vi "HandleObservationSync_003.vi"(8 "error in (no error)":errorcluster, 11 "S4GUI in":refnum<class "S4GUI.lvclass">) -> (0 "error out":errorcluster, 3 "S4GUI out":refnum<class "S4GUI.lvclass">)   [LabVIEW 2018, in "S4GUI.lvclass"] (continued)
          n499 = call-dynamic "Read Channel.vi"("error in (no error)"=w1285, "Acquisition in"=w1286) -> ("error out"=w1268:errorcluster, "Channel.lvclass"=w1267:refnum<class "Channel.lvclass">, "Acquisition out"=w1295:refnum<class "Acquisition.lvclass">)  [unwired: 7 in]
          n500 = call-dynamic "Read Interface.vi"("error in (no error)"=w1268, "Channel in"=w1267) -> ("error out"=w1266:errorcluster, "Interface.lvclass"=w1272:refnum<class "Interface.lvclass">, "Channel out"=w1271:refnum<class "Channel.lvclass">)  [unwired: 7 in]
          n501 = call-dynamic "Get CCD_Config.vi"("error in (no error)"=w1266, "Interface in"=w1272) -> ("error out"=w1279:errorcluster, "output cluster"=w1281:T1, "Interface out"=w1278:refnum<class "Interface.lvclass">)  [unwired: 7 in]
          n502 = Bundle By Name(cluster=w1281, "TRIGGER_MODE"=w1280) -> (w1277:T1)
          n503 = call-dynamic "Set CCD_Config.vi"("error in (no error)"=w1279, "input cluster"=w1277, "Interface in"=w1278) -> ("error out"=w1275:errorcluster, "Interface out"=w1273:refnum<class "Interface.lvclass">)  [unwired: 7 in]
          n504 = Flatten To String(anything=w1277, error in (no error)=w1275) -> (data string=w1276:string, error out=w1274:errorcluster)  [unwired: 2 in, 1 out]
          n505 = call "Write flatted cluster.vi"("error in (no error)"=w1274, "flatted cluster"=w1276, "Interface in"=w1273) -> ("error out"=w1269:errorcluster, "Interface out"=w1270:refnum<class "Interface.lvclass">)  [unwired: 7 in]
          n506 = Increment(x=w1306) -> (x+1=w1305:u32)
          n507 = call-dynamic "Write Interface.vi"("error in (no error)"=w1269, "Interface.lvclass"=w1270, "Channel in"=w1271) -> ("error out"=w1265:errorcluster, "Channel out"=w1264:refnum<class "Channel.lvclass">)  [unwired: 7 in]
          n508 = call-dynamic "Read State Machine.vi"("error in (no error)"=w1265, "Device in"=w1264) -> ("error out"=w1292:errorcluster, "State Machine.lvclass"=w1294:refnum<class "State Machine.lvclass">, "Device out"=w1290:refnum<class "Channel.lvclass">)  [unwired: 7 in]
          n509 = call "Next State.vi"("error in (no error)"=w1292, "New_State"=60, "State Machine in"=w1294) -> ("error out"=w1287:errorcluster, "State Machine out"=w1288:refnum<class "State Machine.lvclass">)  [unwired: 7 in]
          n510 = call-dynamic "Write State Machine.vi"("error in (no error)"=w1287, "State Machine.lvclass"=w1288, "Device in"=w1290) -> ("error out"=w1289:errorcluster, "Device out"=w1291:refnum<class "Channel.lvclass">)  [unwired: 7 in]
          n511 = call-dynamic "Write Channel.vi"("error in (no error)"=w1289, "Channel.lvclass"=w1291, "Acquisition in"=w1295) -> ("error out"=w1282:errorcluster, "Acquisition out"=w1283:refnum<class "Acquisition.lvclass">)  [unwired: 7 in]
          n512 = call-dynamic "Write AcquisitionA.vi"("error in (no error)"=w1282, "Acquisition.lvclass"=w1283, "S4ACS_GUI in"=w1284) -> ("error out"=w1297:errorcluster, "S4ACS_GUI out"=w1296:refnum<class "S4GUI.lvclass">)  [unwired: 7 in]
          n513 = Bundle By Name(cluster=w1296, "Obs_state"=w1305) -> (w1304:refnum<class "S4GUI.lvclass">)
        }
        frame 254 {
          # "Espera terminar a execução do comando atual \nantes de ir ao proximo passo da Observação."
          n514 = call-dynamic "Read AcquisitionA.vi"("error in (no error)"=w1326, "S4ACS_GUI in"=w1327) -> ("error out"=w1332:errorcluster, "Acquisition.lvclass"=w1333:refnum<class "Acquisition.lvclass">, "S4ACS_GUI out"=w1329:refnum<class "S4GUI.lvclass">)  [unwired: 7 in]
          n515 = call-dynamic "Read Channel.vi"("error in (no error)"=w1332, "Acquisition in"=w1333) -> ("error out"=w1324:errorcluster, "Channel.lvclass"=w1323:refnum<class "Channel.lvclass">, "Acquisition out"=w1331:refnum<class "Acquisition.lvclass">)  [unwired: 7 in]
          n516 = call-dynamic "Read State Machine.vi"("error in (no error)"=w1324, "Device in"=w1323) -> ("error out"=w1315:errorcluster, "State Machine.lvclass"=w1317:refnum<class "State Machine.lvclass">, "Device out"=w1321:refnum<class "Channel.lvclass">)  [unwired: 7 in]
          n517 = call-dynamic "Read State.vi"("error in (no error)"=w1315, "State Machine in"=w1317) -> ("error out"=w1314:errorcluster, "State"=w1311:i32, "State Machine out"=w1316:refnum<class "State Machine.lvclass">)  [unwired: 7 in]
          n518 = Equal To 0?(x=w1311) -> (x = 0?=w1313:bool)
          n519 = call-dynamic "Write State Machine.vi"("error in (no error)"=w1314, "State Machine.lvclass"=w1316, "Device in"=w1321) -> ("error out"=w1320:errorcluster, "Device out"=w1322:refnum<class "Channel.lvclass">)  [unwired: 7 in]
          n520 = call-dynamic "Write Channel.vi"("error in (no error)"=w1320, "Channel.lvclass"=w1322, "Acquisition in"=w1331) -> ("error out"=w1328:errorcluster, "Acquisition out"=w1330:refnum<class "Acquisition.lvclass">)  [unwired: 7 in]
          n521 = disable-structure shown="Enabled" {
            disable-tunnel: [u32 299 ("t") w1335] -> w1310
            disable-tunnel: w1309 -> [_ w1336]
            frame Disabled {
            }
            frame Enabled {
              n522 = Increment(x=w1336) -> (x+1=w1335:u32)
            }
          }
          n523 = Select(t=w1310, s=w1313, f=w1309) -> (s? t:f=w1312:u32)
          n524 = call-dynamic "Write AcquisitionA.vi"("error in (no error)"=w1328, "Acquisition.lvclass"=w1330, "S4ACS_GUI in"=w1329) -> ("error out"=w1325:errorcluster, "S4ACS_GUI out"=w1319:refnum<class "S4GUI.lvclass">)  [unwired: 7 in]
          n525 = Bundle By Name(cluster=w1319, "Obs_state"=w1312) -> (w1318:refnum<class "S4GUI.lvclass">)
        }
        frame 255 {
          n526 = call "Read AcquisitionB.vi"("error in (no error)"=w1347, "S4ACS_GUI in"=w1348) -> ("error out"=w1340:errorcluster, "Acquisition.lvclass"=w1341:refnum<class "Acquisition.lvclass">, "S4ACS_GUI out"=w1350:refnum<class "S4GUI.lvclass">)  [unwired: 7 in]
          n527 = call "Read connection.vi"("error in (no error)"=w1340, "Server in"=w1341) -> ("error out"=w1339:errorcluster, "connection"=w1337:bool, "Server out"=w1338:refnum<class "Acquisition.lvclass">)  [unwired: 7 in]
          n528 = case shown="False" w1337 {
            tunnel: w1338 -> [w1358 w1378]
            tunnel: w1339 -> [w1357 w1377]
            tunnel: [w1358 w1375] -> w1351
            tunnel: [w1357 w1374] -> w1349
            tunnel: w1344 -> [w1356 w1367]
            tunnel: [w1352 w1366] -> w1343
            frame False {
              n529 = Increment(x=w1356) -> (x+1=w1355:u32)
              n530 = Increment(x=w1355) -> (x+1=w1354:u32)
              n531 = Increment(x=w1354) -> (x+1=w1353:u32)
              n532 = Increment(x=w1353) -> (x+1=w1352:u32)
            }
            frame True {
              # "configura o canal,\nmas não dispara\na exposicao."
              n533 = call-dynamic "Read Channel.vi"("error in (no error)"=w1377, "Acquisition in"=w1378) -> ("error out"=w1363:errorcluster, "Channel.lvclass"=w1365:refnum<class "Channel.lvclass">, "Acquisition out"=w1376:refnum<class "Acquisition.lvclass">)  [unwired: 7 in]
              n534 = call-dynamic "Write expose.vi"("error in (no error)"=w1363, "expose"=FALSE, "Channel in"=w1365) -> ("error out"=w1362:errorcluster, "Channel out"=w1364:refnum<class "Channel.lvclass">)  [unwired: 7 in]
              n535 = call-dynamic "Read State Machine.vi"("error in (no error)"=w1362, "Device in"=w1364) -> ("error out"=w1371:errorcluster, "State Machine.lvclass"=w1373:refnum<class "State Machine.lvclass">, "Device out"=w1369:refnum<class "Channel.lvclass">)  [unwired: 7 in]
              n536 = call "Next State.vi"("error in (no error)"=w1371, "New_State"=1, "State Machine in"=w1373) -> ("error out"=w1359:errorcluster, "State Machine out"=w1360:refnum<class "State Machine.lvclass">)  [unwired: 7 in]
              n537 = Increment(x=w1367) -> (x+1=w1366:u32)
              n538 = call-dynamic "Write State Machine.vi"("error in (no error)"=w1359, "State Machine.lvclass"=w1360, "Device in"=w1369) -> ("error out"=w1368:errorcluster, "Device out"=w1370:refnum<class "Channel.lvclass">)  [unwired: 7 in]
              n539 = call-dynamic "Write Channel.vi"("error in (no error)"=w1368, "Channel.lvclass"=w1370, "Acquisition in"=w1376) -> ("error out"=w1374:errorcluster, "Acquisition out"=w1375:refnum<class "Acquisition.lvclass">)  [unwired: 7 in]
            }
          }
          n540 = call "Write AcquisitionB.vi"("error in (no error)"=w1349, "Acquisition.lvclass"=w1351, "S4ACS_GUI in"=w1350) -> ("error out"=w1346:errorcluster, "S4ACS_GUI out"=w1345:refnum<class "S4GUI.lvclass">)  [unwired: 7 in]
          n541 = Bundle By Name(cluster=w1345, "Obs_state"=w1343) -> (w1342:refnum<class "S4GUI.lvclass">)
        }
        frame 256 {
          # "Espera terminar a execução do comando atual \nantes de ir ao proximo passo da Observação."
          n542 = call "Read AcquisitionB.vi"("error in (no error)"=w1396, "S4ACS_GUI in"=w1397) -> ("error out"=w1402:errorcluster, "Acquisition.lvclass"=w1403:refnum<class "Acquisition.lvclass">, "S4ACS_GUI out"=w1399:refnum<class "S4GUI.lvclass">)  [unwired: 7 in]
          n543 = call-dynamic "Read Channel.vi"("error in (no error)"=w1402, "Acquisition in"=w1403) -> ("error out"=w1394:errorcluster, "Channel.lvclass"=w1393:refnum<class "Channel.lvclass">, "Acquisition out"=w1401:refnum<class "Acquisition.lvclass">)  [unwired: 7 in]
          n544 = call-dynamic "Read State Machine.vi"("error in (no error)"=w1394, "Device in"=w1393) -> ("error out"=w1385:errorcluster, "State Machine.lvclass"=w1387:refnum<class "State Machine.lvclass">, "Device out"=w1391:refnum<class "Channel.lvclass">)  [unwired: 7 in]
          n545 = call-dynamic "Read State.vi"("error in (no error)"=w1385, "State Machine in"=w1387) -> ("error out"=w1384:errorcluster, "State"=w1381:i32, "State Machine out"=w1386:refnum<class "State Machine.lvclass">)  [unwired: 7 in]
          n546 = call-dynamic "Write State Machine.vi"("error in (no error)"=w1384, "State Machine.lvclass"=w1386, "Device in"=w1391) -> ("error out"=w1390:errorcluster, "Device out"=w1392:refnum<class "Channel.lvclass">)  [unwired: 7 in]
          n547 = call-dynamic "Write Channel.vi"("error in (no error)"=w1390, "Channel.lvclass"=w1392, "Acquisition in"=w1401) -> ("error out"=w1398:errorcluster, "Acquisition out"=w1400:refnum<class "Acquisition.lvclass">)  [unwired: 7 in]
          n548 = Equal To 0?(x=w1381) -> (x = 0?=w1383:bool)
          n549 = disable-structure shown="Enabled" {
            disable-tunnel: [u32 299 ("t") w1405] -> w1379
            disable-tunnel: w1380 -> [_ w1408]
            frame Disabled {
            }
            frame Enabled {
              n550 = Increment(x=w1408) -> (x+1=w1407:u32)
              n551 = Increment(x=w1407) -> (x+1=w1406:u32)
              n552 = Increment(x=w1406) -> (x+1=w1405:u32)
            }
          }
          n553 = Select(t=w1379, s=w1383, f=w1380) -> (s? t:f=w1382:u32)
          n554 = call "Write AcquisitionB.vi"("error in (no error)"=w1398, "Acquisition.lvclass"=w1400, "S4ACS_GUI in"=w1399) -> ("error out"=w1395:errorcluster, "S4ACS_GUI out"=w1389:refnum<class "S4GUI.lvclass">)  [unwired: 7 in]
          n555 = Bundle By Name(cluster=w1389, "Obs_state"=w1382) -> (w1388:refnum<class "S4GUI.lvclass">)
        }
        frame 257 {
          # "Sem SyncBox, \ntrigger mode = 0 (internal)\nCom SyncBox\ntrigger mode = 6 (ext. start)"
          n556 = call-dynamic "Read Sync Box.lvclass.vi"("error in (no error)"=w1446, "SPARC4_AC in"=w1445) -> ("error out"=w1448:errorcluster, "Sync Box.lvclass"=w1449:refnum<class "Sync Box.lvclass">, "SPARC4_AC out"=w1444:refnum<class "S4GUI.lvclass">)  [unwired: 7 in]
          n557 = call "Read connection.vi"("error in (no error)"=w1448, "Server in"=w1449) -> ("error out"=w1447:errorcluster, "connection"=w1410:bool)  [unwired: 7 in, 1 out]
          n558 = case shown="False" w1410 {
            tunnel: [u8 6 ("TRIGGER_MODE") u8 0 ("TRIGGER_MODE")] -> w1409
            frame True {
            }
            frame False {
            }
          }
          n559 = call "Read AcquisitionB.vi"("error in (no error)"=w1447, "S4ACS_GUI in"=w1444) -> ("error out"=w1431:errorcluster, "Acquisition.lvclass"=w1432:refnum<class "Acquisition.lvclass">, "S4ACS_GUI out"=w1430:refnum<class "S4GUI.lvclass">)  [unwired: 7 in]
          n560 = call-dynamic "Read Channel.vi"("error in (no error)"=w1431, "Acquisition in"=w1432) -> ("error out"=w1415:errorcluster, "Channel.lvclass"=w1414:refnum<class "Channel.lvclass">, "Acquisition out"=w1441:refnum<class "Acquisition.lvclass">)  [unwired: 7 in]
          n561 = call-dynamic "Read Interface.vi"("error in (no error)"=w1415, "Channel in"=w1414) -> ("error out"=w1413:errorcluster, "Interface.lvclass"=w1419:refnum<class "Interface.lvclass">, "Channel out"=w1418:refnum<class "Channel.lvclass">)  [unwired: 7 in]
          n562 = call-dynamic "Get CCD_Config.vi"("error in (no error)"=w1413, "Interface in"=w1419) -> ("error out"=w1426:errorcluster, "output cluster"=w1427:T1, "Interface out"=w1425:refnum<class "Interface.lvclass">)  [unwired: 7 in]
          n563 = Bundle By Name(cluster=w1427, "TRIGGER_MODE"=w1409) -> (w1424:T1)
          n564 = call-dynamic "Set CCD_Config.vi"("error in (no error)"=w1426, "input cluster"=w1424, "Interface in"=w1425) -> ("error out"=w1422:errorcluster, "Interface out"=w1420:refnum<class "Interface.lvclass">)  [unwired: 7 in]
          n565 = Flatten To String(anything=w1424, error in (no error)=w1422) -> (data string=w1423:string, error out=w1421:errorcluster)  [unwired: 2 in, 1 out]
          n566 = call "Write flatted cluster.vi"("error in (no error)"=w1421, "flatted cluster"=w1423, "Interface in"=w1420) -> ("error out"=w1416:errorcluster, "Interface out"=w1417:refnum<class "Interface.lvclass">)  [unwired: 7 in]
          n567 = Increment(x=w1452) -> (x+1=w1451:u32)
          n568 = call-dynamic "Write Interface.vi"("error in (no error)"=w1416, "Interface.lvclass"=w1417, "Channel in"=w1418) -> ("error out"=w1412:errorcluster, "Channel out"=w1411:refnum<class "Channel.lvclass">)  [unwired: 7 in]
          n569 = call-dynamic "Read State Machine.vi"("error in (no error)"=w1412, "Device in"=w1411) -> ("error out"=w1438:errorcluster, "State Machine.lvclass"=w1440:refnum<class "State Machine.lvclass">, "Device out"=w1436:refnum<class "Channel.lvclass">)  [unwired: 7 in]
          n570 = call "Next State.vi"("error in (no error)"=w1438, "New_State"=60, "State Machine in"=w1440) -> ("error out"=w1433:errorcluster, "State Machine out"=w1434:refnum<class "State Machine.lvclass">)  [unwired: 7 in]
          n571 = call-dynamic "Write State Machine.vi"("error in (no error)"=w1433, "State Machine.lvclass"=w1434, "Device in"=w1436) -> ("error out"=w1435:errorcluster, "Device out"=w1437:refnum<class "Channel.lvclass">)  [unwired: 7 in]
          n572 = call-dynamic "Write Channel.vi"("error in (no error)"=w1435, "Channel.lvclass"=w1437, "Acquisition in"=w1441) -> ("error out"=w1428:errorcluster, "Acquisition out"=w1429:refnum<class "Acquisition.lvclass">)  [unwired: 7 in]
          n573 = call "Write AcquisitionB.vi"("error in (no error)"=w1428, "Acquisition.lvclass"=w1429, "S4ACS_GUI in"=w1430) -> ("error out"=w1443:errorcluster, "S4ACS_GUI out"=w1442:refnum<class "S4GUI.lvclass">)  [unwired: 7 in]
          n574 = Bundle By Name(cluster=w1442, "Obs_state"=w1451) -> (w1450:refnum<class "S4GUI.lvclass">)
        }
        frame 258 {
          # "Espera terminar a execução do comando atual \nantes de ir ao proximo passo da Observação."
          n575 = call "Read AcquisitionB.vi"("error in (no error)"=w1472, "S4ACS_GUI in"=w1473) -> ("error out"=w1478:errorcluster, "Acquisition.lvclass"=w1479:refnum<class "Acquisition.lvclass">, "S4ACS_GUI out"=w1475:refnum<class "S4GUI.lvclass">)  [unwired: 7 in]
          n576 = call-dynamic "Read Channel.vi"("error in (no error)"=w1478, "Acquisition in"=w1479) -> ("error out"=w1470:errorcluster, "Channel.lvclass"=w1469:refnum<class "Channel.lvclass">, "Acquisition out"=w1477:refnum<class "Acquisition.lvclass">)  [unwired: 7 in]
          n577 = call-dynamic "Read State Machine.vi"("error in (no error)"=w1470, "Device in"=w1469) -> ("error out"=w1461:errorcluster, "State Machine.lvclass"=w1463:refnum<class "State Machine.lvclass">, "Device out"=w1467:refnum<class "Channel.lvclass">)  [unwired: 7 in]
          n578 = call-dynamic "Read State.vi"("error in (no error)"=w1461, "State Machine in"=w1463) -> ("error out"=w1460:errorcluster, "State"=w1457:i32, "State Machine out"=w1462:refnum<class "State Machine.lvclass">)  [unwired: 7 in]
          n579 = call-dynamic "Write State Machine.vi"("error in (no error)"=w1460, "State Machine.lvclass"=w1462, "Device in"=w1467) -> ("error out"=w1466:errorcluster, "Device out"=w1468:refnum<class "Channel.lvclass">)  [unwired: 7 in]
          n580 = call-dynamic "Write Channel.vi"("error in (no error)"=w1466, "Channel.lvclass"=w1468, "Acquisition in"=w1477) -> ("error out"=w1474:errorcluster, "Acquisition out"=w1476:refnum<class "Acquisition.lvclass">)  [unwired: 7 in]
          n581 = Equal To 0?(x=w1457) -> (x = 0?=w1459:bool)
          n582 = Increment(x=w1456) -> (x+1=w1455:u32)
          n583 = Select(t=w1455, s=w1459, f=w1456) -> (s? t:f=w1458:u32)
          n584 = call "Write AcquisitionB.vi"("error in (no error)"=w1474, "Acquisition.lvclass"=w1476, "S4ACS_GUI in"=w1475) -> ("error out"=w1471:errorcluster, "S4ACS_GUI out"=w1465:refnum<class "S4GUI.lvclass">)  [unwired: 7 in]
          n585 = Bundle By Name(cluster=w1465, "Obs_state"=w1458) -> (w1464:refnum<class "S4GUI.lvclass">)
        }
        frame 259 {
          n586 = call-dynamic "Read AcquisitionC.vi"("error in (no error)"=w1490, "S4ACS_GUI in"=w1491) -> ("error out"=w1482:errorcluster, "Acquisition.lvclass"=w1484:refnum<class "Acquisition.lvclass">, "S4ACS_GUI out"=w1493:refnum<class "S4GUI.lvclass">)  [unwired: 7 in]
          n587 = call "Read connection.vi"("error in (no error)"=w1482, "Server in"=w1484) -> ("error out"=w1481:errorcluster, "connection"=w1480:bool, "Server out"=w1483:refnum<class "Acquisition.lvclass">)  [unwired: 7 in]
          n588 = case shown="True" w1480 {
            tunnel: w1483 -> [w1500 w1521]
            tunnel: w1481 -> [w1501 w1520]
            tunnel: [w1500 w1518] -> w1494
            tunnel: [w1501 w1517] -> w1492
            tunnel: w1487 -> [w1499 w1510]
            tunnel: [w1495 w1509] -> w1486
            frame False {
              n589 = Increment(x=w1499) -> (x+1=w1498:u32)
              n590 = Increment(x=w1498) -> (x+1=w1497:u32)
              n591 = Increment(x=w1497) -> (x+1=w1496:u32)
              n592 = Increment(x=w1496) -> (x+1=w1495:u32)
            }
            frame True {
              # "configura o canal,\nmas não dispara\na exposicao."
              n593 = call-dynamic "Read Channel.vi"("error in (no error)"=w1520, "Acquisition in"=w1521) -> ("error out"=w1506:errorcluster, "Channel.lvclass"=w1508:refnum<class "Channel.lvclass">, "Acquisition out"=w1519:refnum<class "Acquisition.lvclass">)  [unwired: 7 in]
              n594 = call-dynamic "Write expose.vi"("error in (no error)"=w1506, "expose"=FALSE, "Channel in"=w1508) -> ("error out"=w1505:errorcluster, "Channel out"=w1507:refnum<class "Channel.lvclass">)  [unwired: 7 in]
              n595 = call-dynamic "Read State Machine.vi"("error in (no error)"=w1505, "Device in"=w1507) -> ("error out"=w1514:errorcluster, "State Machine.lvclass"=w1516:refnum<class "State Machine.lvclass">, "Device out"=w1512:refnum<class "Channel.lvclass">)  [unwired: 7 in]
              n596 = call "Next State.vi"("error in (no error)"=w1514, "New_State"=1, "State Machine in"=w1516) -> ("error out"=w1502:errorcluster, "State Machine out"=w1503:refnum<class "State Machine.lvclass">)  [unwired: 7 in]
              n597 = Increment(x=w1510) -> (x+1=w1509:u32)
              n598 = call-dynamic "Write State Machine.vi"("error in (no error)"=w1502, "State Machine.lvclass"=w1503, "Device in"=w1512) -> ("error out"=w1511:errorcluster, "Device out"=w1513:refnum<class "Channel.lvclass">)  [unwired: 7 in]
              n599 = call-dynamic "Write Channel.vi"("error in (no error)"=w1511, "Channel.lvclass"=w1513, "Acquisition in"=w1519) -> ("error out"=w1517:errorcluster, "Acquisition out"=w1518:refnum<class "Acquisition.lvclass">)  [unwired: 7 in]
            }
          }
          n600 = call-dynamic "Write AcquisitionC.vi"("error in (no error)"=w1492, "Acquisition.lvclass"=w1494, "S4ACS_GUI in"=w1493) -> ("error out"=w1489:errorcluster, "S4ACS_GUI out"=w1488:refnum<class "S4GUI.lvclass">)  [unwired: 7 in]
          n601 = Bundle By Name(cluster=w1488, "Obs_state"=w1486) -> (w1485:refnum<class "S4GUI.lvclass">)
        }
        frame 260 {
          # "Espera terminar a execução do comando atual \nantes de ir ao proximo passo da Observação."
          n602 = call-dynamic "Read AcquisitionC.vi"("error in (no error)"=w1539, "S4ACS_GUI in"=w1540) -> ("error out"=w1545:errorcluster, "Acquisition.lvclass"=w1546:refnum<class "Acquisition.lvclass">, "S4ACS_GUI out"=w1542:refnum<class "S4GUI.lvclass">)  [unwired: 7 in]
          n603 = call-dynamic "Read Channel.vi"("error in (no error)"=w1545, "Acquisition in"=w1546) -> ("error out"=w1537:errorcluster, "Channel.lvclass"=w1536:refnum<class "Channel.lvclass">, "Acquisition out"=w1544:refnum<class "Acquisition.lvclass">)  [unwired: 7 in]
          n604 = call-dynamic "Read State Machine.vi"("error in (no error)"=w1537, "Device in"=w1536) -> ("error out"=w1528:errorcluster, "State Machine.lvclass"=w1530:refnum<class "State Machine.lvclass">, "Device out"=w1534:refnum<class "Channel.lvclass">)  [unwired: 7 in]
          n605 = call-dynamic "Read State.vi"("error in (no error)"=w1528, "State Machine in"=w1530) -> ("error out"=w1527:errorcluster, "State"=w1524:i32, "State Machine out"=w1529:refnum<class "State Machine.lvclass">)  [unwired: 7 in]
          n606 = Equal To 0?(x=w1524) -> (x = 0?=w1526:bool)
          n607 = call-dynamic "Write State Machine.vi"("error in (no error)"=w1527, "State Machine.lvclass"=w1529, "Device in"=w1534) -> ("error out"=w1533:errorcluster, "Device out"=w1535:refnum<class "Channel.lvclass">)  [unwired: 7 in]
          n608 = call-dynamic "Write Channel.vi"("error in (no error)"=w1533, "Channel.lvclass"=w1535, "Acquisition in"=w1544) -> ("error out"=w1541:errorcluster, "Acquisition out"=w1543:refnum<class "Acquisition.lvclass">)  [unwired: 7 in]
          n609 = disable-structure shown="Enabled" {
            disable-tunnel: [u32 299 ("t") w1548] -> w1522
            disable-tunnel: w1523 -> [_ w1551]
            frame Disabled {
            }
            frame Enabled {
              n610 = Increment(x=w1551) -> (x+1=w1550:u32)
              n611 = Increment(x=w1550) -> (x+1=w1549:u32)
              n612 = Increment(x=w1549) -> (x+1=w1548:u32)
            }
          }
          n613 = Select(t=w1522, s=w1526, f=w1523) -> (s? t:f=w1525:u32)
          n614 = call-dynamic "Write AcquisitionC.vi"("error in (no error)"=w1541, "Acquisition.lvclass"=w1543, "S4ACS_GUI in"=w1542) -> ("error out"=w1538:errorcluster, "S4ACS_GUI out"=w1532:refnum<class "S4GUI.lvclass">)  [unwired: 7 in]
          n615 = Bundle By Name(cluster=w1532, "Obs_state"=w1525) -> (w1531:refnum<class "S4GUI.lvclass">)
        }
        frame 261 {
          # "Sem SyncBox, \ntrigger mode = 0 (internal)\nCom SyncBox\ntrigger mode = 6 (ext. start)"
          n616 = call-dynamic "Read Sync Box.lvclass.vi"("error in (no error)"=w1589, "SPARC4_AC in"=w1588) -> ("error out"=w1591:errorcluster, "Sync Box.lvclass"=w1592:refnum<class "Sync Box.lvclass">, "SPARC4_AC out"=w1587:refnum<class "S4GUI.lvclass">)  [unwired: 7 in]
          n617 = call "Read connection.vi"("error in (no error)"=w1591, "Server in"=w1592) -> ("error out"=w1590:errorcluster, "connection"=w1553:bool)  [unwired: 7 in, 1 out]
          n618 = case shown="False" w1553 {
            tunnel: [u8 6 ("TRIGGER_MODE") u8 0 ("TRIGGER_MODE")] -> w1552
            frame True {
            }
            frame False {
            }
          }
          n619 = call-dynamic "Read AcquisitionC.vi"("error in (no error)"=w1590, "S4ACS_GUI in"=w1587) -> ("error out"=w1574:errorcluster, "Acquisition.lvclass"=w1575:refnum<class "Acquisition.lvclass">, "S4ACS_GUI out"=w1573:refnum<class "S4GUI.lvclass">)  [unwired: 7 in]
          n620 = call-dynamic "Read Channel.vi"("error in (no error)"=w1574, "Acquisition in"=w1575) -> ("error out"=w1558:errorcluster, "Channel.lvclass"=w1557:refnum<class "Channel.lvclass">, "Acquisition out"=w1584:refnum<class "Acquisition.lvclass">)  [unwired: 7 in]
          n621 = call-dynamic "Read Interface.vi"("error in (no error)"=w1558, "Channel in"=w1557) -> ("error out"=w1556:errorcluster, "Interface.lvclass"=w1562:refnum<class "Interface.lvclass">, "Channel out"=w1561:refnum<class "Channel.lvclass">)  [unwired: 7 in]
          n622 = call-dynamic "Get CCD_Config.vi"("error in (no error)"=w1556, "Interface in"=w1562) -> ("error out"=w1569:errorcluster, "output cluster"=w1570:T1, "Interface out"=w1568:refnum<class "Interface.lvclass">)  [unwired: 7 in]
          n623 = Bundle By Name(cluster=w1570, "TRIGGER_MODE"=w1552) -> (w1567:T1)
          n624 = call-dynamic "Set CCD_Config.vi"("error in (no error)"=w1569, "input cluster"=w1567, "Interface in"=w1568) -> ("error out"=w1565:errorcluster, "Interface out"=w1563:refnum<class "Interface.lvclass">)  [unwired: 7 in]
          n625 = Flatten To String(anything=w1567, error in (no error)=w1565) -> (data string=w1566:string, error out=w1564:errorcluster)  [unwired: 2 in, 1 out]
          n626 = call "Write flatted cluster.vi"("error in (no error)"=w1564, "flatted cluster"=w1566, "Interface in"=w1563) -> ("error out"=w1559:errorcluster, "Interface out"=w1560:refnum<class "Interface.lvclass">)  [unwired: 7 in]
          n627 = Increment(x=w1595) -> (x+1=w1594:u32)
          n628 = call-dynamic "Write Interface.vi"("error in (no error)"=w1559, "Interface.lvclass"=w1560, "Channel in"=w1561) -> ("error out"=w1555:errorcluster, "Channel out"=w1554:refnum<class "Channel.lvclass">)  [unwired: 7 in]
          n629 = call-dynamic "Read State Machine.vi"("error in (no error)"=w1555, "Device in"=w1554) -> ("error out"=w1581:errorcluster, "State Machine.lvclass"=w1583:refnum<class "State Machine.lvclass">, "Device out"=w1579:refnum<class "Channel.lvclass">)  [unwired: 7 in]
          n630 = call "Next State.vi"("error in (no error)"=w1581, "New_State"=60, "State Machine in"=w1583) -> ("error out"=w1576:errorcluster, "State Machine out"=w1577:refnum<class "State Machine.lvclass">)  [unwired: 7 in]
          n631 = call-dynamic "Write State Machine.vi"("error in (no error)"=w1576, "State Machine.lvclass"=w1577, "Device in"=w1579) -> ("error out"=w1578:errorcluster, "Device out"=w1580:refnum<class "Channel.lvclass">)  [unwired: 7 in]
          n632 = call-dynamic "Write Channel.vi"("error in (no error)"=w1578, "Channel.lvclass"=w1580, "Acquisition in"=w1584) -> ("error out"=w1571:errorcluster, "Acquisition out"=w1572:refnum<class "Acquisition.lvclass">)  [unwired: 7 in]
          n633 = call-dynamic "Write AcquisitionC.vi"("error in (no error)"=w1571, "Acquisition.lvclass"=w1572, "S4ACS_GUI in"=w1573) -> ("error out"=w1586:errorcluster, "S4ACS_GUI out"=w1585:refnum<class "S4GUI.lvclass">)  [unwired: 7 in]
          n634 = Bundle By Name(cluster=w1585, "Obs_state"=w1594) -> (w1593:refnum<class "S4GUI.lvclass">)
        }
        frame 262 {
          # "Espera terminar a execução do comando atual \nantes de ir ao proximo passo da Observação."
          n635 = call-dynamic "Read AcquisitionC.vi"("error in (no error)"=w1615, "S4ACS_GUI in"=w1616) -> ("error out"=w1621:errorcluster, "Acquisition.lvclass"=w1622:refnum<class "Acquisition.lvclass">, "S4ACS_GUI out"=w1618:refnum<class "S4GUI.lvclass">)  [unwired: 7 in]
          n636 = call-dynamic "Read Channel.vi"("error in (no error)"=w1621, "Acquisition in"=w1622) -> ("error out"=w1613:errorcluster, "Channel.lvclass"=w1612:refnum<class "Channel.lvclass">, "Acquisition out"=w1620:refnum<class "Acquisition.lvclass">)  [unwired: 7 in]
          n637 = call-dynamic "Read State Machine.vi"("error in (no error)"=w1613, "Device in"=w1612) -> ("error out"=w1604:errorcluster, "State Machine.lvclass"=w1606:refnum<class "State Machine.lvclass">, "Device out"=w1610:refnum<class "Channel.lvclass">)  [unwired: 7 in]
          n638 = call-dynamic "Read State.vi"("error in (no error)"=w1604, "State Machine in"=w1606) -> ("error out"=w1603:errorcluster, "State"=w1600:i32, "State Machine out"=w1605:refnum<class "State Machine.lvclass">)  [unwired: 7 in]
          n639 = Equal To 0?(x=w1600) -> (x = 0?=w1602:bool)
          n640 = call-dynamic "Write State Machine.vi"("error in (no error)"=w1603, "State Machine.lvclass"=w1605, "Device in"=w1610) -> ("error out"=w1609:errorcluster, "Device out"=w1611:refnum<class "Channel.lvclass">)  [unwired: 7 in]
          n641 = call-dynamic "Write Channel.vi"("error in (no error)"=w1609, "Channel.lvclass"=w1611, "Acquisition in"=w1620) -> ("error out"=w1617:errorcluster, "Acquisition out"=w1619:refnum<class "Acquisition.lvclass">)  [unwired: 7 in]
          n642 = Increment(x=w1599) -> (x+1=w1598:u32)
          n643 = Select(t=w1598, s=w1602, f=w1599) -> (s? t:f=w1601:u32)
          n644 = call-dynamic "Write AcquisitionC.vi"("error in (no error)"=w1617, "Acquisition.lvclass"=w1619, "S4ACS_GUI in"=w1618) -> ("error out"=w1614:errorcluster, "S4ACS_GUI out"=w1608:refnum<class "S4GUI.lvclass">)  [unwired: 7 in]
          n645 = Bundle By Name(cluster=w1608, "Obs_state"=w1601) -> (w1607:refnum<class "S4GUI.lvclass">)
        }
        frame 263 {
          # "Dispara o comando para o dispositivo corrente."
          n646 = call-dynamic "Read AcquisitionD.vi"("error in (no error)"=w1633, "S4ACS_GUI in"=w1634) -> ("error out"=w1626:errorcluster, "Acquisition.lvclass"=w1627:refnum<class "Acquisition.lvclass">, "S4ACS_GUI out"=w1636:refnum<class "S4GUI.lvclass">)  [unwired: 7 in]
          n647 = call "Read connection.vi"("error in (no error)"=w1626, "Server in"=w1627) -> ("error out"=w1624:errorcluster, "connection"=w1623:bool, "Server out"=w1625:refnum<class "Acquisition.lvclass">)  [unwired: 7 in]
          n648 = case shown="True" w1623 {
            tunnel: w1625 -> [w1640 w1660]
            tunnel: w1624 -> [w1639 w1659]
            tunnel: [w1640 w1657] -> w1637
            tunnel: [w1639 w1656] -> w1635
            tunnel: w1630 -> [_ w1649]
            tunnel: [u32 299 w1648] -> w1629
            frame False {
            }
            frame True {
              # "configura o canal,\nmas não dispara\na exposicao."
              n649 = call-dynamic "Read Channel.vi"("error in (no error)"=w1659, "Acquisition in"=w1660) -> ("error out"=w1645:errorcluster, "Channel.lvclass"=w1647:refnum<class "Channel.lvclass">, "Acquisition out"=w1658:refnum<class "Acquisition.lvclass">)  [unwired: 7 in]
              n650 = call-dynamic "Write expose.vi"("error in (no error)"=w1645, "expose"=FALSE, "Channel in"=w1647) -> ("error out"=w1644:errorcluster, "Channel out"=w1646:refnum<class "Channel.lvclass">)  [unwired: 7 in]
              n651 = call-dynamic "Read State Machine.vi"("error in (no error)"=w1644, "Device in"=w1646) -> ("error out"=w1653:errorcluster, "State Machine.lvclass"=w1655:refnum<class "State Machine.lvclass">, "Device out"=w1651:refnum<class "Channel.lvclass">)  [unwired: 7 in]
              n652 = call "Next State.vi"("error in (no error)"=w1653, "New_State"=1, "State Machine in"=w1655) -> ("error out"=w1641:errorcluster, "State Machine out"=w1642:refnum<class "State Machine.lvclass">)  [unwired: 7 in]
              n653 = Increment(x=w1649) -> (x+1=w1648:u32)
              n654 = call-dynamic "Write State Machine.vi"("error in (no error)"=w1641, "State Machine.lvclass"=w1642, "Device in"=w1651) -> ("error out"=w1650:errorcluster, "Device out"=w1652:refnum<class "Channel.lvclass">)  [unwired: 7 in]
              n655 = call-dynamic "Write Channel.vi"("error in (no error)"=w1650, "Channel.lvclass"=w1652, "Acquisition in"=w1658) -> ("error out"=w1656:errorcluster, "Acquisition out"=w1657:refnum<class "Acquisition.lvclass">)  [unwired: 7 in]
            }
          }
          n656 = call-dynamic "Write AcquisitionD.vi"("error in (no error)"=w1635, "Acquisition.lvclass"=w1637, "S4ACS_GUI in"=w1636) -> ("error out"=w1632:errorcluster, "S4ACS_GUI out"=w1631:refnum<class "S4GUI.lvclass">)  [unwired: 7 in]
          n657 = Bundle By Name(cluster=w1631, "Obs_state"=w1629) -> (w1628:refnum<class "S4GUI.lvclass">)
        }
        frame 264 {
          # "Espera terminar a execução do comando atual \nantes de ir ao proximo passo da Observação."
          n658 = call-dynamic "Read AcquisitionD.vi"("error in (no error)"=w1678, "S4ACS_GUI in"=w1679) -> ("error out"=w1684:errorcluster, "Acquisition.lvclass"=w1685:refnum<class "Acquisition.lvclass">, "S4ACS_GUI out"=w1681:refnum<class "S4GUI.lvclass">)  [unwired: 7 in]
          n659 = call-dynamic "Read Channel.vi"("error in (no error)"=w1684, "Acquisition in"=w1685) -> ("error out"=w1676:errorcluster, "Channel.lvclass"=w1675:refnum<class "Channel.lvclass">, "Acquisition out"=w1683:refnum<class "Acquisition.lvclass">)  [unwired: 7 in]
          n660 = call-dynamic "Read State Machine.vi"("error in (no error)"=w1676, "Device in"=w1675) -> ("error out"=w1667:errorcluster, "State Machine.lvclass"=w1669:refnum<class "State Machine.lvclass">, "Device out"=w1673:refnum<class "Channel.lvclass">)  [unwired: 7 in]
          n661 = call-dynamic "Read State.vi"("error in (no error)"=w1667, "State Machine in"=w1669) -> ("error out"=w1666:errorcluster, "State"=w1663:i32, "State Machine out"=w1668:refnum<class "State Machine.lvclass">)  [unwired: 7 in]
          n662 = Equal To 0?(x=w1663) -> (x = 0?=w1665:bool)
          n663 = call-dynamic "Write State Machine.vi"("error in (no error)"=w1666, "State Machine.lvclass"=w1668, "Device in"=w1673) -> ("error out"=w1672:errorcluster, "Device out"=w1674:refnum<class "Channel.lvclass">)  [unwired: 7 in]
          n664 = call-dynamic "Write Channel.vi"("error in (no error)"=w1672, "Channel.lvclass"=w1674, "Acquisition in"=w1683) -> ("error out"=w1680:errorcluster, "Acquisition out"=w1682:refnum<class "Acquisition.lvclass">)  [unwired: 7 in]
          n665 = disable-structure shown="Enabled" {
            disable-tunnel: w1662 -> [w1687 _]
            disable-tunnel: [w1686 u32 299] -> w1661
            frame Disabled {
              n666 = Increment(x=w1687) -> (x+1=w1686:u32)
            }
            frame Enabled {
            }
          }
          n667 = Select(t=w1661, s=w1665, f=w1662) -> (s? t:f=w1664:u32)
          n668 = call-dynamic "Write AcquisitionD.vi"("error in (no error)"=w1680, "Acquisition.lvclass"=w1682, "S4ACS_GUI in"=w1681) -> ("error out"=w1677:errorcluster, "S4ACS_GUI out"=w1671:refnum<class "S4GUI.lvclass">)  [unwired: 7 in]
          n669 = Bundle By Name(cluster=w1671, "Obs_state"=w1664) -> (w1670:refnum<class "S4GUI.lvclass">)
        }
        frame 265 {
          # "Sem SyncBox, \ntrigger mode = 0 (internal)\nCom SyncBox\ntrigger mode = 6 (ext. start)"
          n670 = call-dynamic "Read Sync Box.lvclass.vi"("error in (no error)"=w1726, "SPARC4_AC in"=w1725) -> ("error out"=w1728:errorcluster, "Sync Box.lvclass"=w1729:refnum<class "Sync Box.lvclass">, "SPARC4_AC out"=w1724:refnum<class "S4GUI.lvclass">)  [unwired: 7 in]
          n671 = call "Read connection.vi"("error in (no error)"=w1728, "Server in"=w1729) -> ("error out"=w1727:errorcluster, "connection"=w1690:bool)  [unwired: 7 in, 1 out]
          n672 = case shown="False" w1690 {
            tunnel: [u8 6 ("TRIGGER_MODE") u8 0 ("TRIGGER_MODE")] -> w1689
            frame True {
            }
            frame False {
            }
          }
          n673 = call-dynamic "Read AcquisitionD.vi"("error in (no error)"=w1727, "S4ACS_GUI in"=w1724) -> ("error out"=w1711:errorcluster, "Acquisition.lvclass"=w1712:refnum<class "Acquisition.lvclass">, "S4ACS_GUI out"=w1710:refnum<class "S4GUI.lvclass">)  [unwired: 7 in]
          n674 = call-dynamic "Read Channel.vi"("error in (no error)"=w1711, "Acquisition in"=w1712) -> ("error out"=w1695:errorcluster, "Channel.lvclass"=w1694:refnum<class "Channel.lvclass">, "Acquisition out"=w1721:refnum<class "Acquisition.lvclass">)  [unwired: 7 in]
          n675 = call-dynamic "Read Interface.vi"("error in (no error)"=w1695, "Channel in"=w1694) -> ("error out"=w1693:errorcluster, "Interface.lvclass"=w1699:refnum<class "Interface.lvclass">, "Channel out"=w1698:refnum<class "Channel.lvclass">)  [unwired: 7 in]
          n676 = call-dynamic "Get CCD_Config.vi"("error in (no error)"=w1693, "Interface in"=w1699) -> ("error out"=w1706:errorcluster, "output cluster"=w1707:T1, "Interface out"=w1705:refnum<class "Interface.lvclass">)  [unwired: 7 in]
          n677 = Bundle By Name(cluster=w1707, "TRIGGER_MODE"=w1689) -> (w1704:T1)
          n678 = call-dynamic "Set CCD_Config.vi"("error in (no error)"=w1706, "input cluster"=w1704, "Interface in"=w1705) -> ("error out"=w1702:errorcluster, "Interface out"=w1700:refnum<class "Interface.lvclass">)  [unwired: 7 in]
          n679 = Flatten To String(anything=w1704, error in (no error)=w1702) -> (data string=w1703:string, error out=w1701:errorcluster)  [unwired: 2 in, 1 out]
          n680 = call "Write flatted cluster.vi"("error in (no error)"=w1701, "flatted cluster"=w1703, "Interface in"=w1700) -> ("error out"=w1696:errorcluster, "Interface out"=w1697:refnum<class "Interface.lvclass">)  [unwired: 7 in]
          n681 = call-dynamic "Write Interface.vi"("error in (no error)"=w1696, "Interface.lvclass"=w1697, "Channel in"=w1698) -> ("error out"=w1692:errorcluster, "Channel out"=w1691:refnum<class "Channel.lvclass">)  [unwired: 7 in]
          n682 = call-dynamic "Read State Machine.vi"("error in (no error)"=w1692, "Device in"=w1691) -> ("error out"=w1718:errorcluster, "State Machine.lvclass"=w1720:refnum<class "State Machine.lvclass">, "Device out"=w1716:refnum<class "Channel.lvclass">)  [unwired: 7 in]
          n683 = Increment(x=w1732) -> (x+1=w1731:u32)
          n684 = call "Next State.vi"("error in (no error)"=w1718, "New_State"=60, "State Machine in"=w1720) -> ("error out"=w1713:errorcluster, "State Machine out"=w1714:refnum<class "State Machine.lvclass">)  [unwired: 7 in]
          n685 = call-dynamic "Write State Machine.vi"("error in (no error)"=w1713, "State Machine.lvclass"=w1714, "Device in"=w1716) -> ("error out"=w1715:errorcluster, "Device out"=w1717:refnum<class "Channel.lvclass">)  [unwired: 7 in]
          n686 = call-dynamic "Write Channel.vi"("error in (no error)"=w1715, "Channel.lvclass"=w1717, "Acquisition in"=w1721) -> ("error out"=w1708:errorcluster, "Acquisition out"=w1709:refnum<class "Acquisition.lvclass">)  [unwired: 7 in]
          n687 = call-dynamic "Write AcquisitionD.vi"("error in (no error)"=w1708, "Acquisition.lvclass"=w1709, "S4ACS_GUI in"=w1710) -> ("error out"=w1723:errorcluster, "S4ACS_GUI out"=w1722:refnum<class "S4GUI.lvclass">)  [unwired: 7 in]
          n688 = Bundle By Name(cluster=w1722, "Obs_state"=w1731) -> (w1730:refnum<class "S4GUI.lvclass">)
        }
        frame 266 {
          # "Espera terminar a execução do comando atual \nantes de ir ao proximo passo da Observação."
          n689 = call-dynamic "Read AcquisitionD.vi"("error in (no error)"=w1752, "S4ACS_GUI in"=w1753) -> ("error out"=w1758:errorcluster, "Acquisition.lvclass"=w1759:refnum<class "Acquisition.lvclass">, "S4ACS_GUI out"=w1755:refnum<class "S4GUI.lvclass">)  [unwired: 7 in]
          n690 = call-dynamic "Read Channel.vi"("error in (no error)"=w1758, "Acquisition in"=w1759) -> ("error out"=w1750:errorcluster, "Channel.lvclass"=w1749:refnum<class "Channel.lvclass">, "Acquisition out"=w1757:refnum<class "Acquisition.lvclass">)  [unwired: 7 in]
          n691 = call-dynamic "Read State Machine.vi"("error in (no error)"=w1750, "Device in"=w1749) -> ("error out"=w1741:errorcluster, "State Machine.lvclass"=w1743:refnum<class "State Machine.lvclass">, "Device out"=w1747:refnum<class "Channel.lvclass">)  [unwired: 7 in]
          n692 = call-dynamic "Read State.vi"("error in (no error)"=w1741, "State Machine in"=w1743) -> ("error out"=w1740:errorcluster, "State"=w1737:i32, "State Machine out"=w1742:refnum<class "State Machine.lvclass">)  [unwired: 7 in]
          n693 = Equal To 0?(x=w1737) -> (x = 0?=w1739:bool)
          n694 = call-dynamic "Write State Machine.vi"("error in (no error)"=w1740, "State Machine.lvclass"=w1742, "Device in"=w1747) -> ("error out"=w1746:errorcluster, "Device out"=w1748:refnum<class "Channel.lvclass">)  [unwired: 7 in]
          n695 = call-dynamic "Write Channel.vi"("error in (no error)"=w1746, "Channel.lvclass"=w1748, "Acquisition in"=w1757) -> ("error out"=w1754:errorcluster, "Acquisition out"=w1756:refnum<class "Acquisition.lvclass">)  [unwired: 7 in]
          n696 = Select(t=u32 299, s=w1739, f=w1736) -> (s? t:f=w1738:u32)
          n697 = call-dynamic "Write AcquisitionD.vi"("error in (no error)"=w1754, "Acquisition.lvclass"=w1756, "S4ACS_GUI in"=w1755) -> ("error out"=w1751:errorcluster, "S4ACS_GUI out"=w1745:refnum<class "S4GUI.lvclass">)  [unwired: 7 in]
          n698 = Bundle By Name(cluster=w1745, "Obs_state"=w1738) -> (w1744:refnum<class "S4GUI.lvclass">)
        }
        frame 271 {
          # "Prepara os canais de aquisição para sequencia de foco...."
          n699 = flat-sequence {
            tunnel: w1786 -> [w1891]
            tunnel: [w1891] -> w1785
            frame #0 {
              n700 = Tick Count (ms)() -> (millisecond timer value=→"time5":u32)
            }
          }
          n701 = call-dynamic "Read AcquisitionA.vi"("error in (no error)"=w1785, "S4ACS_GUI in"=w1807) -> ("error out"=w1805:errorcluster, "Acquisition.lvclass"=w1806:refnum<class "Acquisition.lvclass">, "S4ACS_GUI out"=w1809:refnum<class "S4GUI.lvclass">)  [unwired: 7 in]
          n702 = call "Read connection.vi"("error in (no error)"=w1805, "Server in"=w1806) -> ("error out"=w1804:errorcluster, "connection"=w1784:bool, "Server out"=w1803:refnum<class "Acquisition.lvclass">)  [unwired: 7 in]
          n703 = case shown="True" w1784 {
            tunnel: [w1872 w1890] -> w1810
            tunnel: [w1871 w1889] -> w1808
            tunnel: w1804 -> [w1871 w1888]
            tunnel: w1803 -> [w1872 w1887]
            frame False {
            }
            frame True {
              # "configura o canal,\nmas não dispara\na exposicao."
              n704 = call-dynamic "Read Channel.vi"("error in (no error)"=w1888, "Acquisition in"=w1887) -> ("error out"=w1877:errorcluster, "Channel.lvclass"=w1879:refnum<class "Channel.lvclass">, "Acquisition out"=w1886:refnum<class "Acquisition.lvclass">)  [unwired: 7 in]
              n705 = call-dynamic "Write expose.vi"("error in (no error)"=w1877, "expose"=FALSE, "Channel in"=w1879) -> ("error out"=w1876:errorcluster, "Channel out"=w1878:refnum<class "Channel.lvclass">)  [unwired: 7 in]
              n706 = call-dynamic "Read State Machine.vi"("error in (no error)"=w1876, "Device in"=w1878) -> ("error out"=w1883:errorcluster, "State Machine.lvclass"=w1885:refnum<class "State Machine.lvclass">, "Device out"=w1881:refnum<class "Channel.lvclass">)  [unwired: 7 in]
              n707 = call "Next State.vi"("error in (no error)"=w1883, "New_State"=1, "State Machine in"=w1885) -> ("error out"=w1873:errorcluster, "State Machine out"=w1874:refnum<class "State Machine.lvclass">)  [unwired: 7 in]
              n708 = call-dynamic "Write State Machine.vi"("error in (no error)"=w1873, "State Machine.lvclass"=w1874, "Device in"=w1881) -> ("error out"=w1880:errorcluster, "Device out"=w1882:refnum<class "Channel.lvclass">)  [unwired: 7 in]
              n709 = call-dynamic "Write Channel.vi"("error in (no error)"=w1880, "Channel.lvclass"=w1882, "Acquisition in"=w1886) -> ("error out"=w1889:errorcluster, "Acquisition out"=w1890:refnum<class "Acquisition.lvclass">)  [unwired: 7 in]
            }
          }
          n710 = Increment(x=w1802) -> (x+1=w1766:u32)
          n711 = call-dynamic "Write AcquisitionA.vi"("error in (no error)"=w1808, "Acquisition.lvclass"=w1810, "S4ACS_GUI in"=w1809) -> ("error out"=w1798:errorcluster, "S4ACS_GUI out"=w1797:refnum<class "S4GUI.lvclass">)  [unwired: 7 in]
          n712 = call "Read AcquisitionB.vi"("error in (no error)"=w1798, "S4ACS_GUI in"=w1797) -> ("error out"=w1799:errorcluster, "Acquisition.lvclass"=w1800:refnum<class "Acquisition.lvclass">, "S4ACS_GUI out"=w1801:refnum<class "S4GUI.lvclass">)  [unwired: 7 in]
          n713 = call "Read connection.vi"("error in (no error)"=w1799, "Server in"=w1800) -> ("error out"=w1782:errorcluster, "connection"=w1781:bool, "Server out"=w1783:refnum<class "Acquisition.lvclass">)  [unwired: 7 in]
          n714 = case shown="True" w1781 {
            tunnel: [w1852 w1870] -> w1780
            tunnel: [w1851 w1869] -> w1779
            tunnel: w1782 -> [w1851 w1868]
            tunnel: w1783 -> [w1852 w1867]
            frame False {
            }
            frame True {
              # "configura o canal,\nmas não dispara\na exposicao."
              n715 = call-dynamic "Read Channel.vi"("error in (no error)"=w1868, "Acquisition in"=w1867) -> ("error out"=w1857:errorcluster, "Channel.lvclass"=w1859:refnum<class "Channel.lvclass">, "Acquisition out"=w1866:refnum<class "Acquisition.lvclass">)  [unwired: 7 in]
              n716 = call-dynamic "Write expose.vi"("error in (no error)"=w1857, "expose"=FALSE, "Channel in"=w1859) -> ("error out"=w1856:errorcluster, "Channel out"=w1858:refnum<class "Channel.lvclass">)  [unwired: 7 in]
              n717 = call-dynamic "Read State Machine.vi"("error in (no error)"=w1856, "Device in"=w1858) -> ("error out"=w1863:errorcluster, "State Machine.lvclass"=w1865:refnum<class "State Machine.lvclass">, "Device out"=w1861:refnum<class "Channel.lvclass">)  [unwired: 7 in]
              n718 = call "Next State.vi"("error in (no error)"=w1863, "New_State"=1, "State Machine in"=w1865) -> ("error out"=w1853:errorcluster, "State Machine out"=w1854:refnum<class "State Machine.lvclass">)  [unwired: 7 in]
              n719 = call-dynamic "Write State Machine.vi"("error in (no error)"=w1853, "State Machine.lvclass"=w1854, "Device in"=w1861) -> ("error out"=w1860:errorcluster, "Device out"=w1862:refnum<class "Channel.lvclass">)  [unwired: 7 in]
              n720 = call-dynamic "Write Channel.vi"("error in (no error)"=w1860, "Channel.lvclass"=w1862, "Acquisition in"=w1866) -> ("error out"=w1869:errorcluster, "Acquisition out"=w1870:refnum<class "Acquisition.lvclass">)  [unwired: 7 in]
            }
          }
          n721 = call "Write AcquisitionB.vi"("error in (no error)"=w1779, "Acquisition.lvclass"=w1780, "S4ACS_GUI in"=w1801) -> ("error out"=w1790:errorcluster, "S4ACS_GUI out"=w1789:refnum<class "S4GUI.lvclass">)  [unwired: 7 in]
          n722 = call-dynamic "Read AcquisitionC.vi"("error in (no error)"=w1790, "S4ACS_GUI in"=w1789) -> ("error out"=w1794:errorcluster, "Acquisition.lvclass"=w1795:refnum<class "Acquisition.lvclass">, "S4ACS_GUI out"=w1796:refnum<class "S4GUI.lvclass">)  [unwired: 7 in]
          n723 = call "Read connection.vi"("error in (no error)"=w1794, "Server in"=w1795) -> ("error out"=w1776:errorcluster, "connection"=w1777:bool, "Server out"=w1778:refnum<class "Acquisition.lvclass">)  [unwired: 7 in]
          n724 = case shown="True" w1777 {
            tunnel: [w1832 w1850] -> w1775
            tunnel: [w1831 w1849] -> w1774
            tunnel: w1776 -> [w1831 w1848]
            tunnel: w1778 -> [w1832 w1847]
            frame False {
            }
            frame True {
              # "configura o canal,\nmas não dispara\na exposicao."
              n725 = call-dynamic "Read Channel.vi"("error in (no error)"=w1848, "Acquisition in"=w1847) -> ("error out"=w1837:errorcluster, "Channel.lvclass"=w1839:refnum<class "Channel.lvclass">, "Acquisition out"=w1846:refnum<class "Acquisition.lvclass">)  [unwired: 7 in]
              n726 = call-dynamic "Write expose.vi"("error in (no error)"=w1837, "expose"=FALSE, "Channel in"=w1839) -> ("error out"=w1836:errorcluster, "Channel out"=w1838:refnum<class "Channel.lvclass">)  [unwired: 7 in]
              n727 = call-dynamic "Read State Machine.vi"("error in (no error)"=w1836, "Device in"=w1838) -> ("error out"=w1843:errorcluster, "State Machine.lvclass"=w1845:refnum<class "State Machine.lvclass">, "Device out"=w1841:refnum<class "Channel.lvclass">)  [unwired: 7 in]
              n728 = call "Next State.vi"("error in (no error)"=w1843, "New_State"=1, "State Machine in"=w1845) -> ("error out"=w1833:errorcluster, "State Machine out"=w1834:refnum<class "State Machine.lvclass">)  [unwired: 7 in]
              n729 = call-dynamic "Write State Machine.vi"("error in (no error)"=w1833, "State Machine.lvclass"=w1834, "Device in"=w1841) -> ("error out"=w1840:errorcluster, "Device out"=w1842:refnum<class "Channel.lvclass">)  [unwired: 7 in]
              n730 = call-dynamic "Write Channel.vi"("error in (no error)"=w1840, "Channel.lvclass"=w1842, "Acquisition in"=w1846) -> ("error out"=w1849:errorcluster, "Acquisition out"=w1850:refnum<class "Acquisition.lvclass">)  [unwired: 7 in]
            }
          }
          n731 = call-dynamic "Write AcquisitionC.vi"("error in (no error)"=w1774, "Acquisition.lvclass"=w1775, "S4ACS_GUI in"=w1796) -> ("error out"=w1788:errorcluster, "S4ACS_GUI out"=w1787:refnum<class "S4GUI.lvclass">)  [unwired: 7 in]
          n732 = call-dynamic "Read AcquisitionD.vi"("error in (no error)"=w1788, "S4ACS_GUI in"=w1787) -> ("error out"=w1791:errorcluster, "Acquisition.lvclass"=w1792:refnum<class "Acquisition.lvclass">, "S4ACS_GUI out"=w1793:refnum<class "S4GUI.lvclass">)  [unwired: 7 in]
          n733 = call "Read connection.vi"("error in (no error)"=w1791, "Server in"=w1792) -> ("error out"=w1771:errorcluster, "connection"=w1773:bool, "Server out"=w1772:refnum<class "Acquisition.lvclass">)  [unwired: 7 in]
          n734 = case shown="True" w1773 {
            tunnel: [w1812 w1830] -> w1770
            tunnel: [w1811 w1829] -> w1769
            tunnel: w1771 -> [w1811 w1828]
            tunnel: w1772 -> [w1812 w1827]
            frame False {
            }
            frame True {
              # "configura o canal,\nmas não dispara\na exposicao."
              n735 = call-dynamic "Read Channel.vi"("error in (no error)"=w1828, "Acquisition in"=w1827) -> ("error out"=w1817:errorcluster, "Channel.lvclass"=w1819:refnum<class "Channel.lvclass">, "Acquisition out"=w1826:refnum<class "Acquisition.lvclass">)  [unwired: 7 in]
              n736 = call-dynamic "Write expose.vi"("error in (no error)"=w1817, "expose"=FALSE, "Channel in"=w1819) -> ("error out"=w1816:errorcluster, "Channel out"=w1818:refnum<class "Channel.lvclass">)  [unwired: 7 in]
              n737 = call-dynamic "Read State Machine.vi"("error in (no error)"=w1816, "Device in"=w1818) -> ("error out"=w1823:errorcluster, "State Machine.lvclass"=w1825:refnum<class "State Machine.lvclass">, "Device out"=w1821:refnum<class "Channel.lvclass">)  [unwired: 7 in]
              n738 = call "Next State.vi"("error in (no error)"=w1823, "New_State"=1, "State Machine in"=w1825) -> ("error out"=w1813:errorcluster, "State Machine out"=w1814:refnum<class "State Machine.lvclass">)  [unwired: 7 in]
              n739 = call-dynamic "Write State Machine.vi"("error in (no error)"=w1813, "State Machine.lvclass"=w1814, "Device in"=w1821) -> ("error out"=w1820:errorcluster, "Device out"=w1822:refnum<class "Channel.lvclass">)  [unwired: 7 in]
              n740 = call-dynamic "Write Channel.vi"("error in (no error)"=w1820, "Channel.lvclass"=w1822, "Acquisition in"=w1826) -> ("error out"=w1829:errorcluster, "Acquisition out"=w1830:refnum<class "Acquisition.lvclass">)  [unwired: 7 in]
            }
          }
          n741 = call-dynamic "Write AcquisitionD.vi"("error in (no error)"=w1769, "Acquisition.lvclass"=w1770, "S4ACS_GUI in"=w1793) -> ("error out"=w1761:errorcluster, "S4ACS_GUI out"=w1765:refnum<class "S4GUI.lvclass">)  [unwired: 7 in]
          n742 = Unbundle By Name(w1765) -> ("TelFocus.lvclass"=w1764:refnum<class "TelFocus.lvclass">)
          n743 = call-dynamic "Write focus #stepsdone.vi"("error in (no error)"=w1761, "focus #stepsdone"=u32 0, "TelFocus in"=w1764) -> ("error out"=w1760:errorcluster, "TelFocus out"=w1762:refnum<class "TelFocus.lvclass">)  [unwired: 7 in]
          n744 = Bundle By Name(cluster=w1765, "TelFocus.lvclass"=w1762, "Error Msg"="", "Obs_state"=w1766) -> (w1767:refnum<class "S4GUI.lvclass">)
        }
        frame 272 {
          w1901 = 38 ("x")
          w1910 = 28 ("x")
          # "Se algum canal foi pra 38: Texp inválido \npara a configuração do CCD."
          # "Se algum canal foi pra 28: ERRO na inicialização."
          # "Espera terminar a execução da preparação\ndos 4 canais antes de ir ao proximo passo \nda Observação."
          n745 = flat-sequence {
            tunnel: w1943 -> [w2048]
            tunnel: [w2048] -> w1942
            frame #0 {
              n746 = Tick Count (ms)() -> (millisecond timer value=→"time6":u32)
            }
          }
          n747 = call-dynamic "Read AcquisitionA.vi"("error in (no error)"=w1942, "S4ACS_GUI in"=w1953) -> ("error out"=w1940:errorcluster, "Acquisition.lvclass"=w1941:refnum<class "Acquisition.lvclass">, "S4ACS_GUI out"=w1955:refnum<class "S4GUI.lvclass">)  [unwired: 7 in]
          n748 = call "Read connection.vi"("error in (no error)"=w1940, "Server in"=w1941) -> ("error out"=w1938:errorcluster, "connection"=w1937:bool, "Server out"=w1939:refnum<class "Acquisition.lvclass">)  [unwired: 7 in]
          n749 = case shown="True" w1937 {
            tunnel: w1939 -> [w2031 w2047]
            tunnel: w1938 -> [w2030 w2046]
            tunnel: [w2031 w2044] -> w1956
            tunnel: [w2030 w2043] -> w1954
            tunnel: [0 ("State") w2033] -> w1900
            frame False {
            }
            frame True {
              n750 = call-dynamic "Read Channel.vi"("error in (no error)"=w2046, "Acquisition in"=w2047) -> ("error out"=w2042:errorcluster, "Channel.lvclass"=w2041:refnum<class "Channel.lvclass">, "Acquisition out"=w2045:refnum<class "Acquisition.lvclass">)  [unwired: 7 in]
              n751 = call-dynamic "Read State Machine.vi"("error in (no error)"=w2042, "Device in"=w2041) -> ("error out"=w2035:errorcluster, "State Machine.lvclass"=w2037:refnum<class "State Machine.lvclass">, "Device out"=w2039:refnum<class "Channel.lvclass">)  [unwired: 7 in]
              n752 = call-dynamic "Read State.vi"("error in (no error)"=w2035, "State Machine in"=w2037) -> ("error out"=w2034:errorcluster, "State"=w2033:i32, "State Machine out"=w2036:refnum<class "State Machine.lvclass">)  [unwired: 7 in]
              n753 = call-dynamic "Write State Machine.vi"("error in (no error)"=w2034, "State Machine.lvclass"=w2036, "Device in"=w2039) -> ("error out"=w2038:errorcluster, "Device out"=w2040:refnum<class "Channel.lvclass">)  [unwired: 7 in]
              n754 = call-dynamic "Write Channel.vi"("error in (no error)"=w2038, "Channel.lvclass"=w2040, "Acquisition in"=w2045) -> ("error out"=w2043:errorcluster, "Acquisition out"=w2044:refnum<class "Acquisition.lvclass">)  [unwired: 7 in]
            }
          }
          n755 = call-dynamic "Write AcquisitionA.vi"("error in (no error)"=w1954, "Acquisition.lvclass"=w1956, "S4ACS_GUI in"=w1955) -> ("error out"=w1950:errorcluster, "S4ACS_GUI out"=w1949:refnum<class "S4GUI.lvclass">)  [unwired: 7 in]
          n756 = call "Read AcquisitionB.vi"("error in (no error)"=w1950, "S4ACS_GUI in"=w1949) -> ("error out"=w1932:errorcluster, "Acquisition.lvclass"=w1935:refnum<class "Acquisition.lvclass">, "S4ACS_GUI out"=w1936:refnum<class "S4GUI.lvclass">)  [unwired: 7 in]
          n757 = call "Read connection.vi"("error in (no error)"=w1932, "Server in"=w1935) -> ("error out"=w1931:errorcluster, "connection"=w1933:bool, "Server out"=w1934:refnum<class "Acquisition.lvclass">)  [unwired: 7 in]
          n758 = case shown="True" w1933 {
            tunnel: w1934 -> [w2013 w2029]
            tunnel: w1931 -> [w2012 w2028]
            tunnel: [w2013 w2026] -> w1930
            tunnel: [w2012 w2025] -> w1929
            tunnel: [0 ("State") w2015] -> w1899
            frame False {
            }
            frame True {
              n759 = call-dynamic "Read Channel.vi"("error in (no error)"=w2028, "Acquisition in"=w2029) -> ("error out"=w2024:errorcluster, "Channel.lvclass"=w2023:refnum<class "Channel.lvclass">, "Acquisition out"=w2027:refnum<class "Acquisition.lvclass">)  [unwired: 7 in]
              n760 = call-dynamic "Read State Machine.vi"("error in (no error)"=w2024, "Device in"=w2023) -> ("error out"=w2017:errorcluster, "State Machine.lvclass"=w2019:refnum<class "State Machine.lvclass">, "Device out"=w2021:refnum<class "Channel.lvclass">)  [unwired: 7 in]
              n761 = call-dynamic "Read State.vi"("error in (no error)"=w2017, "State Machine in"=w2019) -> ("error out"=w2016:errorcluster, "State"=w2015:i32, "State Machine out"=w2018:refnum<class "State Machine.lvclass">)  [unwired: 7 in]
              n762 = call-dynamic "Write State Machine.vi"("error in (no error)"=w2016, "State Machine.lvclass"=w2018, "Device in"=w2021) -> ("error out"=w2020:errorcluster, "Device out"=w2022:refnum<class "Channel.lvclass">)  [unwired: 7 in]
              n763 = call-dynamic "Write Channel.vi"("error in (no error)"=w2020, "Channel.lvclass"=w2022, "Acquisition in"=w2027) -> ("error out"=w2025:errorcluster, "Acquisition out"=w2026:refnum<class "Acquisition.lvclass">)  [unwired: 7 in]
            }
          }
          n764 = call "Write AcquisitionB.vi"("error in (no error)"=w1929, "Acquisition.lvclass"=w1930, "S4ACS_GUI in"=w1936) -> ("error out"=w1948:errorcluster, "S4ACS_GUI out"=w1947:refnum<class "S4GUI.lvclass">)  [unwired: 7 in]
